vi "PIEZO_read_position.vi"(6 "MCL Handle":i32, 7 "Autofocus ON?":bool, 8 "error MCL in":errorcluster, 9 "Reset":bool, 11 "Autofocus cluster":T1) -> (0 "error MCL out":errorcluster, 1 "Autofocus cluster OUT":T1, 2 "Z piezo":dbl, 3 "Stable?":bool)   [LabVIEW 2015]
uses:
  <vilib>/Analysis/baseanly.llb/Mean (DBL).vi
  <userlib>/Madlib.dll
  <vilib>/Analysis/NI_AALBase.lvlib
panel:
  out "Piezo chart":dbl(graph)
  out "dz/dt":dbl format="%0.3f"
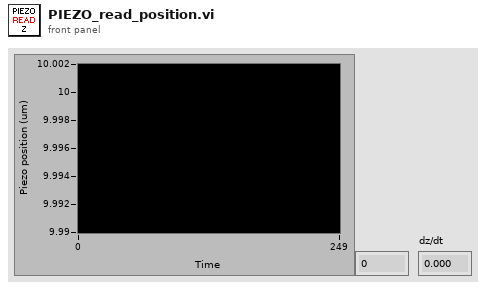
[diagram p1: front panel]
types:
  T1 = cluster{"Setpoint":dbl, "Ref channel":bool, "dimension size":i32, "X_derivation":dbl[], "Y_derivation":dbl[], "Slope":dbl, "iteration":i32, "PID gains":cluster{"proportional gain (Kc)":dbl, "integral time (Ti, min)":dbl, "derivative time (Td, min)":dbl}, "z0":dbl, "Switch":bool, "Autocalibration":bool, "Init":bool, "i IR lost":i32, "Derivation array":dbl[], "QPDcount":u32}
  T2 = enum16{"Always On", "Always Off", "Off While Running"}
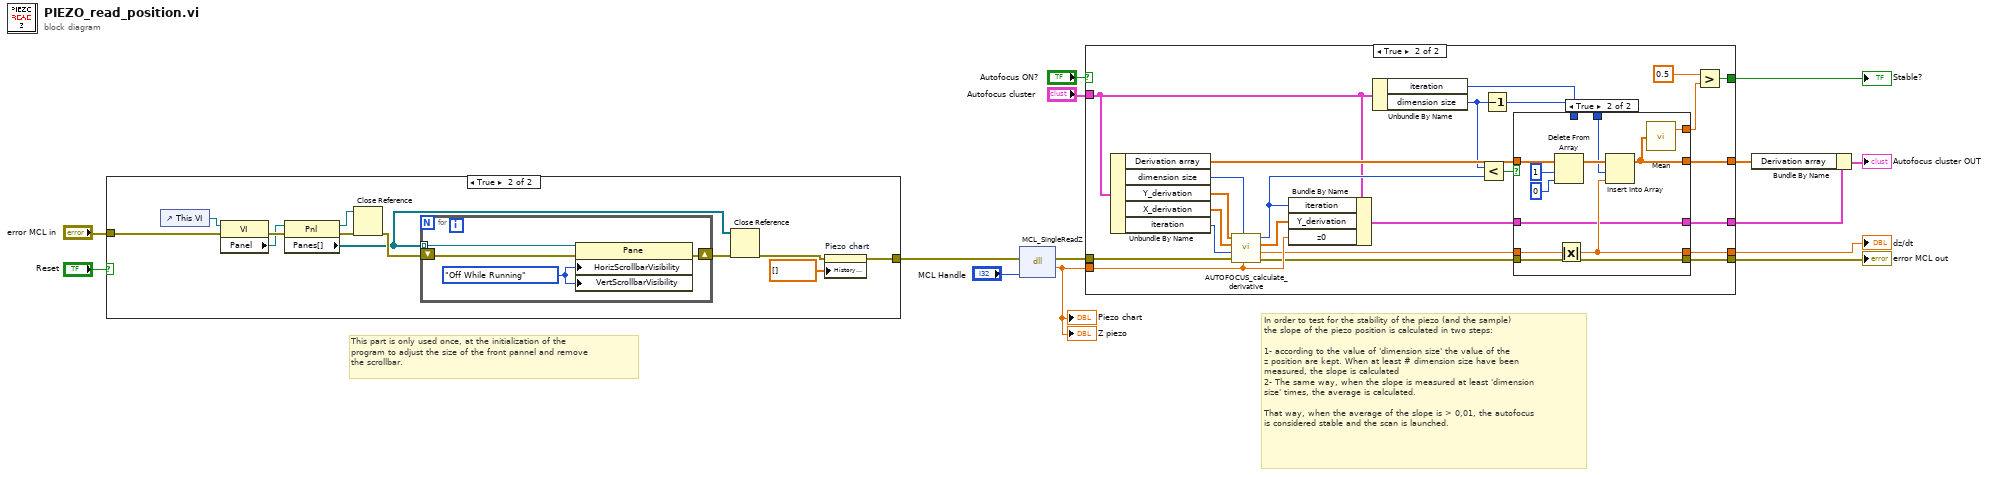
[diagram p0: block diagram]
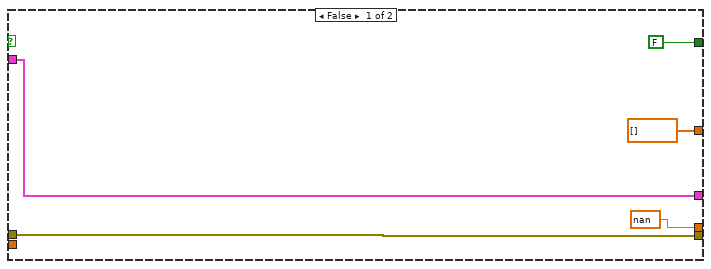
[diagram p2: hidden frame]
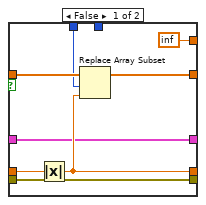
[diagram p3: hidden frame]
diagram:
  # "In order to test for the stability of the piezo (and the sample)\nthe slope of the piezo position is calculated in two steps:\n\n1- according to the value of 'dimension size' the value of the\nz position are kept. When at least # dimension size have been\nmeasured, the slope is calculated\n2- The same way, when the slope is measured at least 'dimension\nsize' times, the average is calculated.\n\nThat way, when the average of the slope is > 0,01, the autofocus\nis considered stable and the scan is launched."
  # "This part is only used once, at the initialization of the \nprogram to adjust the size of the front pannel and remove\nthe scrollbar."
  n1 = case shown="True" "Reset" {
    tunnel: "error MCL in" -> [w15 w17]
    tunnel: [w15 w27] -> w11
    frame False {
    }
    frame True {
      n2 = control-ref of="This VI"() -> (w18:refnum<vi>)
      n3 = property class="VI"(reference=w18, error in=w17) -> (error out=w20:errorcluster, "Panel"=w19:refnum<vi>)  [unwired: 1 out]
      n4 = property class="Pnl"(reference=w19, error in=w20) -> (reference out=w21:refnum<vi>, error out=w22:errorcluster, "Panes[]"=w24:refnum<vi>[])
      n5 = Close Reference(reference=w21, error in (no error)=w22) -> (error out=w25:errorcluster)
      n6 = for {
        tunnel: w24 -> [w31] mode=indexing
        shift-right: [w29] -> w23
        shift-left: w25 -> [w28]
        w30 = T2."Off While Running" ("Horizontal Scrollbar Visibility")
        n7 = property class="Pane"(reference=w31, error in=w28, "HorizScrollbarVisibility"=w30, "VertScrollbarVisibility"=w30) -> (error out=w29:errorcluster)  [unwired: 1 out]
      }
      n8 = Close Reference(reference=w24, error in (no error)=w23) -> (error out=w16:errorcluster)
      n9 = property on="Piezo chart" class="WFChart (strict)"(error in=w16, "History Data"=dbl[] []) -> (error out=w27:errorcluster)  [unwired: 1 in, 1 out]
    }
  }
  n10 = dll-call lib="C:/Program Files/National Instruments/LabVIEW 2015/user.lib/Madlib.dll" fn="MCL_SingleReadZ"(error in=w11, "Handle"="MCL Handle") -> (error out=w9:errorcluster, "Z"=w8:dbl)  [unwired: 3 in, 1 out]
  "Z piezo" <- w8
  "Piezo chart" <- w8
  n11 = case shown="True" "Autofocus ON?" {
    tunnel: w9 -> [w36 w60]
    tunnel: w8 -> [_ w55]
    tunnel: [w36 w40] -> w7
    tunnel: [nan ("dx/dt") w44] -> w6
    tunnel: [FALSE w53] -> w5
    tunnel: "Autofocus cluster" -> [w33 w48]
    tunnel: [dbl[] [] ("Derivation array") w38] -> w3
    tunnel: [w33 w37] -> w4
    frame False {
    }
    frame True {
      n12 = Unbundle By Name(w48) -> ("Derivation array"=w49:dbl[], "dimension size"=w51:i32, "Y_derivation"=w57:dbl[], "X_derivation"=w58:dbl[], "iteration"=w59:i32)
      n13 = call "AUTOFOCUS_calculate_derivative.vi"("z"=w55, "Dimension size"=w51, "error in"=w60, "iteration"=w59, "X"=w58, "Y"=w57) -> ("error out"=w41:errorcluster, "dx/dt"=w45:dbl, "Y out"=w56:dbl[], "iteration out"=w52:i32)
      n14 = Bundle By Name(cluster=w48, "iteration"=w52, "Y_derivation"=w56, "z0"=w55) -> (w39:T1)
      n15 = Unbundle By Name(w48) -> ("iteration"=w42:i32, "dimension size"=w46:i32)
      n16 = Less?(x=w46, y=w52) -> (x < y?=w50:bool)
      n17 = Decrement(x=w46) -> (x-1=w47:i32)
      n18 = case shown="True" w50 {
        tunnel: w49 -> [w67 w79]
        tunnel: w45 -> [w68 w74]
        tunnel: w47 -> [_ w75]
        tunnel: [w66 w73] -> w44
        tunnel: [inf w72] -> w43
        tunnel: w42 -> [w65 _]
        tunnel: w41 -> [w63 w71]
        tunnel: [w63 w71] -> w40
        tunnel: w39 -> [w62 w70]
        tunnel: [w62 w70] -> w37
        tunnel: [w61 w69] -> w38
        frame False {
          n19 = Absolute Value(x=w68) -> (abs(x)=w66:dbl)
          n20 = Replace Array Subset(array=w67, new element=w66, index=w65) -> (w61:dbl[])
        }
        frame True {
          n21 = Delete From Array(array=w79, length=1, index=0) -> (array with subset deleted=w76:dbl[])  [unwired: 1 out]
          n22 = Absolute Value(x=w74) -> (abs(x)=w73:dbl)
          n23 = Insert Into Array(array=w76, index=w75, new element=w73) -> (w69:dbl[])
          n24 = call-poly <vilib>:"Mean.vi"("X"=w69) -> ("mean"=w72:dbl)  [unwired: 1 out]
        }
      }
      n25 = Greater?(x=0.5, y=w43) -> (0:w53:bool)
    }
  }
  "error MCL out" <- w7
  "dz/dt" <- w6
  "Stable?" <- w5
  n26 = Bundle By Name(cluster=w4, "Derivation array"=w3) -> (→"Autofocus cluster OUT":T1)
